vi "Parametric Curve Fit.vi"() -> ()   [LabVIEW 2023]
doc: "This VI uses the Fitting VIs to fit equations to curves and calculate confidence intervals.\n\nYou must select <B>Least Square</B> as the fitting <B>Method</B> to calculate the confidence interval of a fitted curve. The <B>Least Absolute Residual</B> and <B>Bisquare</B> fitting methods are less sensitive to outliers than the <B>Least Square</B> fitting method."
uses:
  <vilib>/Analysis/6fits.llb/Confidence Interval (Linear).vi
  <vilib>/Analysis/6fits.llb/Confidence Interval (Exp).vi
  <vilib>/Analysis/6fits.llb/Confidence Interval (Power).vi
  <vilib>/Analysis/6fits.llb/Confidence Interval (Gauss).vi
  <vilib>/Analysis/6fits.llb/Confidence Interval (Log).vi
  <vilib>/Analysis/NI_AALPro.lvlib
panel:
  in  "Intercept":string="Intercept"
  in  "Slope":string="Slope"
  in  "Scale":string="Scale"
  in  "Center":string="Center"
  in  "Power":string="Power"
  in  "Damping":string="Damping"
  in  "Amplitude":string="Amplitude"
  in  "Stop":bool
  out "Residue":dbl
  in  "Add outliers?":bool
  out "Slope Value":dbl format="%#.6g"
  out "Intercept Value":dbl format="%#.6g"
  in  "Tolerance":dbl=0.0001
  in  "Fitting Method":u16(ring) items=["Least Square", "Least Absolute Residual", "Bisquare"]
  in  "Data Set":T1(ring)
  out "Standard Deviation":dbl
  out "Observed Data and Fitted Curve":cluster{cluster{dbl, "Numeric":dbl}[]}[](graph)
  # "Overview: Demonstrates the use of the Advanced Curve Fitting VIs for determining the confidence interval of a best fit curve.\nRequirements: LabVIEW Full Development System\nInstructions:\n1. Run the VI. \n2. Select the Data Set and Fitting Method and view the results.\n3. Click Stop to stop the VI."
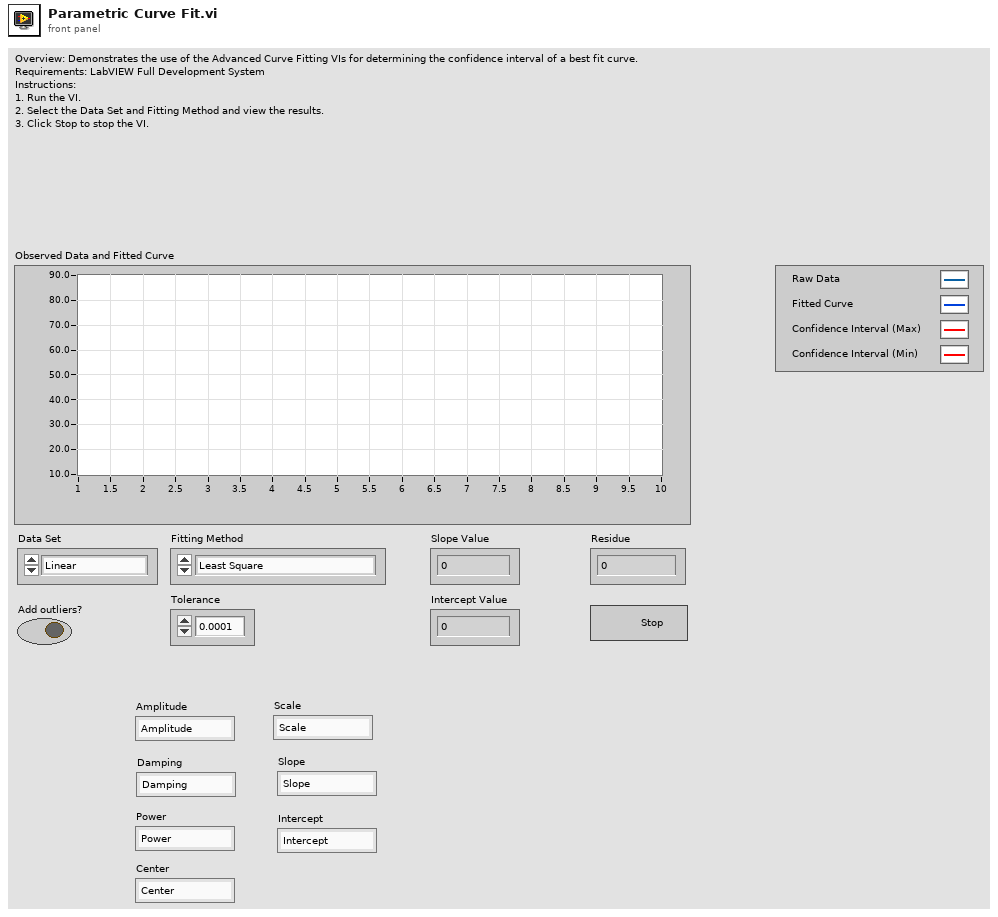
[diagram p1: front panel]
types:
  T1 = enum16{"Linear", "Exponential", "Power", "Gaussian", "Logarithmic"}
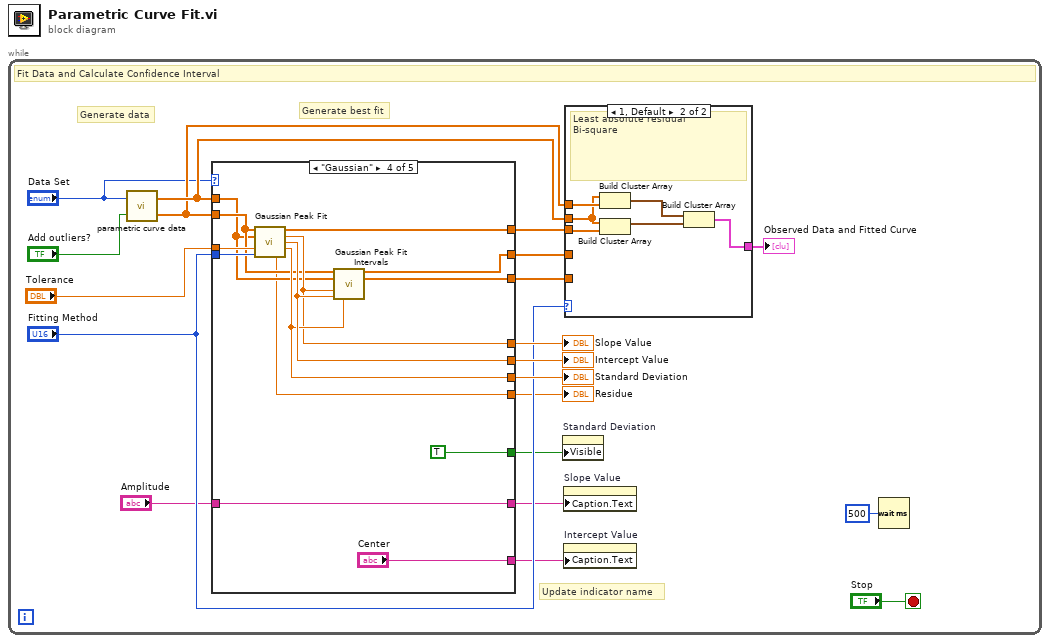
[diagram p0: block diagram]
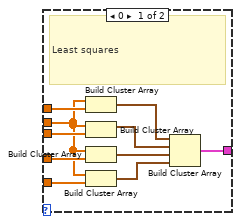
[diagram p2: hidden frame]
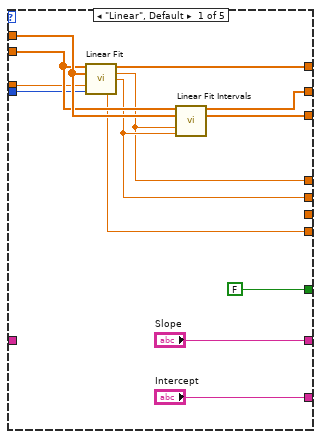
[diagram p3: hidden frame]
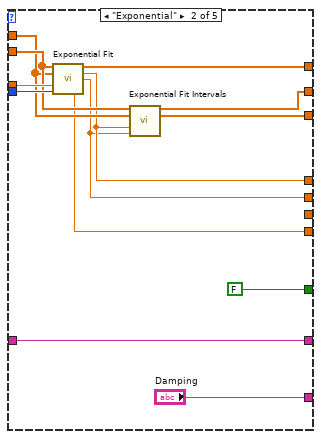
[diagram p4: hidden frame]
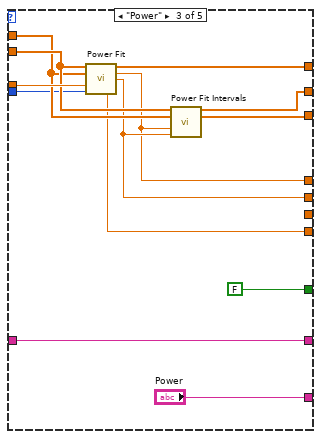
[diagram p5: hidden frame]
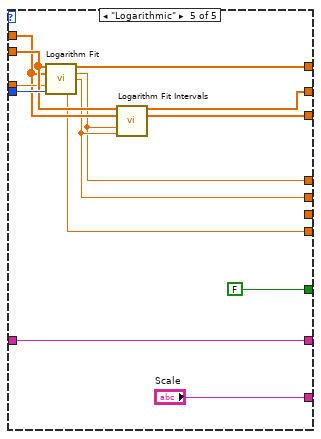
[diagram p6: hidden frame]
diagram:
  n1 = while {
    stop <- "Stop" stop-if-true
    # "Update indicator name"
    # "Generate best fit"
    # "Generate data"
    # "Fit Data and Calculate Confidence Interval"
    n2 = call "parametric curve data.vi"("Add outliers?"="Add outliers?", "Signal type"="Data Set") -> ("Y"=w15:dbl[], "X"=w16:dbl[])
    n3 = case shown="\"Gaussian\"" "Data Set" {
      tunnel: [w49 w56 w72 w86 w100] -> w17
      tunnel: [w48 w57 w70 w87 w102] -> w19
      tunnel: [w47 w58 w71 w88 w101] -> w18
      tunnel: w16 -> [w46 w59 w73 w80 w96]
      tunnel: w15 -> [w45 w60 w74 w81 w98]
      tunnel: "Tolerance" -> [w44 w62 w75 w89 w97]
      tunnel: "Fitting Method" -> [w43 w61 w69 w85 w99]
      tunnel: [w42 w54 w68 w84 w95] -> w13
      tunnel: [w40 w55 w67 w82 w94] -> w14
      tunnel: [_ _ _ w83 _] -> w12
      tunnel: [w41 w53 w66 w79 w93] -> w7
      tunnel: ["Intercept" "Damping" "Power" "Center" "Scale"] -> w4
      tunnel: ["Slope" w51 w64 w77 w91] -> w3
      tunnel: [FALSE ("Visible") FALSE ("Visible") FALSE ("Visible") TRUE ("Visible") FALSE ("Visible")] -> w2
      tunnel: "Amplitude" -> [_ w51 w64 w77 w91]
      frame "Linear", Default {
        n4 = call <vilib>:"Linear Fit.vi"("Y"=w45, "X"=w46, "tolerance"=w44, "method"=w43) -> ("Best Linear Fit"=w49:dbl[], "slope"=w40:dbl, "intercept"=w42:dbl, "residue"=w41:dbl)  [unwired: 7 in, 1 out]
        n5 = call-poly <vilib>:"Linear Fit Intervals.vi"("Y"=w45, "X"=w46, "slope"=w40, "intercept"=w42) -> ("Upper Bound"=w47:dbl[], "Lower Bound"=w48:dbl[])  [unwired: 7 in, 3 out]
      }
      frame "Exponential" {
        n6 = call <vilib>:"Exponential Fit.vi"("Y"=w60, "X"=w59, "tolerance"=w62, "method"=w61) -> ("Best Exponential Fit"=w56:dbl[], "amplitude"=w55:dbl, "damping"=w54:dbl, "residue"=w53:dbl)  [unwired: 6 in, 2 out]
        n7 = call-poly <vilib>:"Exponential Fit Intervals.vi"("Y"=w60, "X"=w59, "amplitude"=w55, "damping"=w54) -> ("Upper Bound"=w58:dbl[], "Lower Bound"=w57:dbl[])  [unwired: 7 in, 3 out]
      }
      frame "Power" {
        n8 = call <vilib>:"Power Fit.vi"("Y"=w74, "X"=w73, "tolerance"=w75, "method"=w69) -> ("Best Power Fit"=w72:dbl[], "amplitude"=w67:dbl, "power"=w68:dbl, "residue"=w66:dbl)  [unwired: 6 in, 2 out]
        n9 = call-poly <vilib>:"Power Fit Intervals.vi"("Y"=w74, "X"=w73, "amplitude"=w67, "power"=w68) -> ("Upper Bound"=w71:dbl[], "Lower Bound"=w70:dbl[])  [unwired: 7 in, 3 out]
      }
      frame "Gaussian" {
        n10 = call <vilib>:"Gaussian Peak Fit.vi"("Y"=w81, "X"=w80, "tolerance"=w89, "method"=w85) -> ("Best Gaussian Fit"=w86:dbl[], "amplitude"=w82:dbl, "center"=w84:dbl, "standard deviation"=w83:dbl, "residue"=w79:dbl)  [unwired: 5 in, 2 out]
        n11 = call-poly <vilib>:"Gaussian Peak Fit Intervals.vi"("Y"=w81, "X"=w80, "amplitude"=w82, "center"=w84, "standard deviation"=w83) -> ("Upper Bound"=w88:dbl[], "Lower Bound"=w87:dbl[])  [unwired: 5 in, 4 out]
      }
      frame "Logarithmic" {
        n12 = call <vilib>:"Logarithm Fit.vi"("Y"=w98, "X"=w96, "tolerance"=w97, "method"=w99) -> ("Best Logarithm Fit"=w100:dbl[], "amplitude"=w94:dbl, "scale"=w95:dbl, "residue"=w93:dbl)  [unwired: 7 in, 1 out]
        n13 = call-poly <vilib>:"Logarithm Fit Intervals.vi"("Y"=w98, "X"=w96, "amplitude"=w94, "scale"=w95) -> ("Upper Bound"=w101:dbl[], "Lower Bound"=w102:dbl[])  [unwired: 7 in, 3 out]
      }
    }
    "Slope Value" <- w14
    "Intercept Value" <- w13
    "Standard Deviation" <- w12
    "Residue" <- w7
    n14 = property on="Standard Deviation" class="DigNum (strict)"("Visible"=w2) -> ()  [unwired: 2 in, 2 out]
    n15 = property on="Slope Value" class="DigNum (strict)"("Caption.Text"=w3) -> ()  [unwired: 2 in, 2 out]
    n16 = property on="Intercept Value" class="DigNum (strict)"("Caption.Text"=w4) -> ()  [unwired: 2 in, 2 out]
    n17 = case shown="1, Default" "Fitting Method" {
      tunnel: w15 -> [w26 w33]
      tunnel: w16 -> [w21 w32]
      tunnel: w19 -> [w25 _]
      tunnel: w18 -> [w24 _]
      tunnel: w17 -> [w23 w34]
      tunnel: [w22 w31] -> w8
      frame 0 {
        # "Least squares"
        n18 = Build Cluster Array(w21, w26) -> (w28:cluster{dbl, dbl}[])
        n19 = Build Cluster Array(w21, w23) -> (w27:cluster{dbl, "Numeric":dbl}[])
        n20 = Build Cluster Array(w21, w24) -> (w30:cluster{dbl, "Numeric":dbl}[])
        n21 = Build Cluster Array(w21, w25) -> (w29:cluster{dbl, "Numeric":dbl}[])
        n22 = Build Cluster Array(w28, w27, w30, w29) -> (w22:cluster{cluster{dbl, "Numeric":dbl}[]}[])
      }
      frame 1, Default {
        # "Least absolute residual\nBi-square"
        n23 = Build Cluster Array(w32, w33) -> (w36:cluster{dbl, dbl}[])
        n24 = Build Cluster Array(w32, w34) -> (w35:cluster{dbl, "Numeric":dbl}[])
        n25 = Build Cluster Array(w36, w35) -> (w31:cluster{cluster{dbl, "Numeric":dbl}[]}[])
      }
    }
    "Observed Data and Fitted Curve" <- w8
    n26 = Wait (ms)(milliseconds to wait=u32 500) -> ()  [unwired: 1 out]
  }
